vi "Get bookmark.vi"(10 "Paths":path[](array[path])) -> (2 "Execute vi Path":path[](array[path]))   [LabVIEW 2019, in "UnitTestEngine.lvlib" / "TestRunner.lvclass"]
uses:
  TestRunner.lvclass
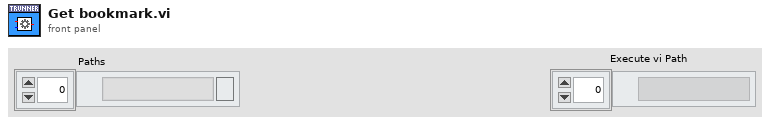
[diagram p1: front panel]
types:
  T1 = typedef "LVBookmarkInfoTypeDef.ctl" = cluster{"Bookmark Reference":u32, "Bookmark Tag":string, "Label Text":string}[]
  T2 = cluster{"Bookmark Reference":u32, "Bookmark Tag":string, "Label Text":string}
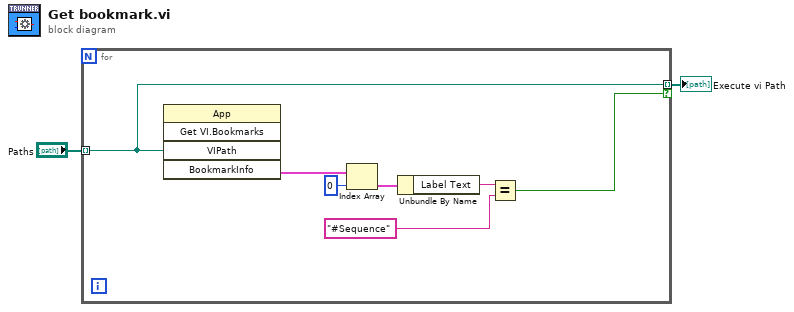
[diagram p0: block diagram]
diagram:
  n1 = for {
    tunnel: "Paths" -> [w4] mode=indexing
    tunnel: [w4] -> w1 mode=indexing if=w3
    n2 = invoke class="App" method="Get VI.Bookmarks"("VIPath"=w4) -> ("BookmarkInfo"=w9:T1)  [unwired: 4 in, 4 out]
    n3 = Index Array(array=w9, index=0) -> (element=w7:T2)
    n4 = Unbundle By Name(w7) -> ("Label Text"=w6:string)
    n5 = Equal?(x=w6, y="#Sequence") -> (x = y?=w3:bool)
  }
  "Execute vi Path" <- w1
